vi "明场校正.vi"() -> ()   [LabVIEW 2018]
uses:
  <vilib>/vision/Process.llb/Surface Fit Options.ctl
  <vilib>/vision/Process.llb/Background Estimation Options.ctl
  <vilib>/vision/NI_Vision_Development_Module.lvlib
panel:
  in  "停止":bool
  out "error out":errorcluster
  out "Image":T1(plugin-control)
  in  "枚举":enum16{"估算", "采集"}(ring)
  in  "Background Estimation Options":T2={"Estimate Background?"=FALSE, "Method"=0, "Polynomial Degree"=2, "Window Size (32x32)"={"SizeX"=32, "SizeY"=32}, "Niblack Deviation Factor (0.2)"=0.2} {"Niblack Deviation Factor (0.2)" min=0.0 max=1.0 format="%.2f"; "Window Size (32x32)"."SizeY" min=3 step=1; "Window Size (32x32)"."SizeX" min=3 step=1; "Method" items=["Polynomial", "Background Correction", "NiBlack"]}
  in  "Surface Fit Options":T3={"Model"=0, "Sampling Grid Size"={"SizeX"=100, "SizeY"=100}, "Polynomial Degree"=2} {"Sampling Grid Size"."SizeY" min=3 step=1; "Sampling Grid Size"."SizeX" min=3 step=1; "Model" items=["Polynomial"]}
  in  "路径":path
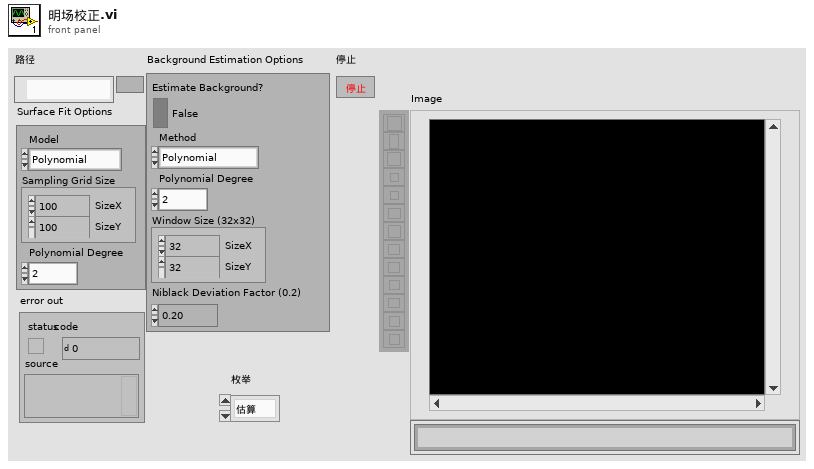
[diagram p1: front panel]
types:
  T1 = typedef "IMAQ Image.ctl" = refnum<image>
  T2 = typedef "Background Estimation Options.ctl" = cluster{"Estimate Background?":bool, "Method":i32, "Polynomial Degree":i32, "Window Size (32x32)":cluster{"SizeX":i32, "SizeY":i32}, "Niblack Deviation Factor (0.2)":dbl}
  T3 = typedef "Surface Fit Options.ctl" = cluster{"Model":i32, "Sampling Grid Size":cluster{"SizeX":i32, "SizeY":i32}, "Polynomial Degree":i32}
  T4 = cluster{"Surface Fit Options":T3, "Background Estimation Options":T2, "枚举":enum16{"估算", "采集"}}
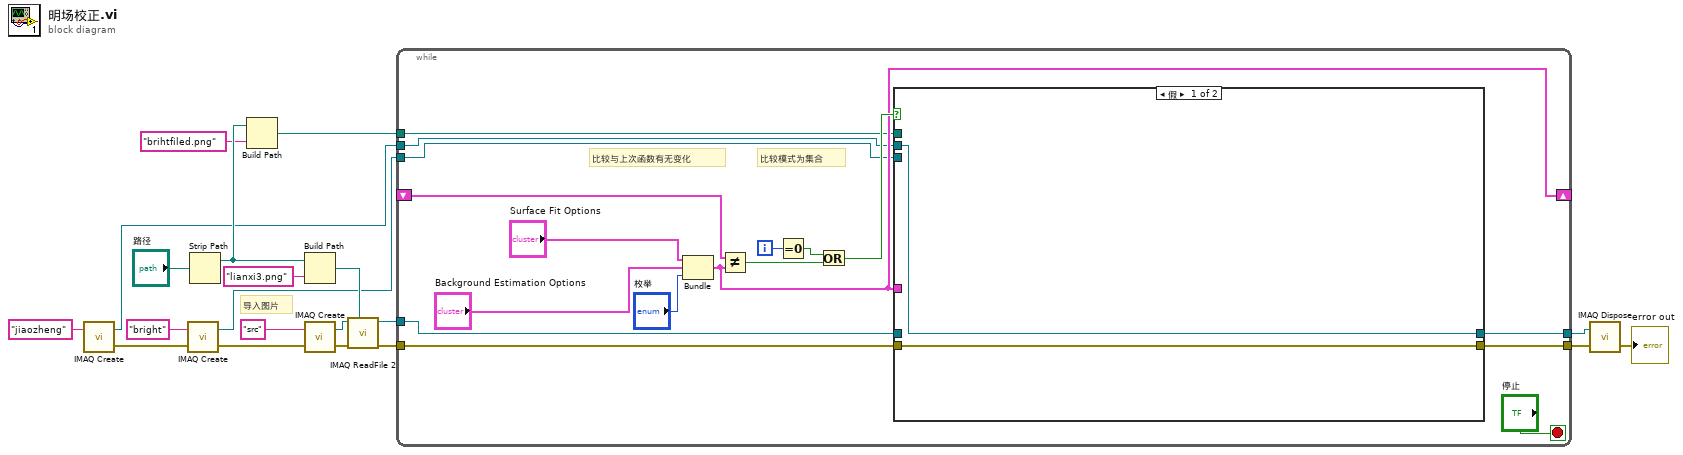
[diagram p0: block diagram]
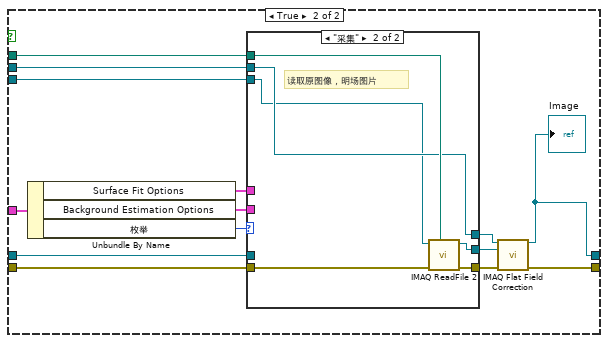
[diagram p2: hidden frame]
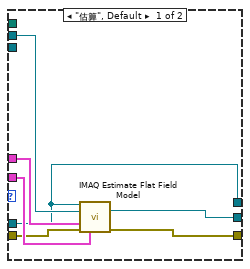
[diagram p3: hidden frame]
diagram:
  # "导入图片"
  n1 = call "IMAQ Create"("Image Name"="jiaozheng") -> ("New Image"=w11:T1, "error out"=w2:errorcluster)  [unwired: 4 in]
  n2 = call "IMAQ Create"("Image Name"="bright", "error in (no error)"=w2) -> ("New Image"=w4:T1, "error out"=w3:errorcluster)  [unwired: 3 in]
  n3 = Strip Path(path="路径") -> (stripped path=w19:path)  [unwired: 1 out]
  n4 = Build Path(base path=w19, name or relative path="brihtfiled.png" ("名称或相对路径")) -> (appended path=w6:path)
  n5 = Build Path(base path=w19, name or relative path="lianxi3.png" ("名称或相对路径")) -> (appended path=w15:path)
  n6 = call "IMAQ Create"("Image Name"="src", "error in (no error)"=w3) -> ("New Image"=w14:T1, "error out"=w13:errorcluster)  [unwired: 3 in]
  n7 = call "IMAQ ReadFile 2"("File Path"=w15, "error in (no error)"=w13, "Image"=w14) -> ("error out"=w10:errorcluster, "Image Out"=w12:T1)  [unwired: 4 in, 3 out]
  n8 = while {
    shift-right: [w29] -> _
    shift-left: _ -> [w34]
    tunnel: w12 -> [w28]
    tunnel: w11 -> [w27]
    tunnel: w10 -> [w26]
    tunnel: [w25] -> w9
    tunnel: [w24] -> w8
    tunnel: w6 -> [w23]
    tunnel: w4 -> [w22]
    i -> [w33]
    stop <- "停止" stop-if-true
    # "比较模式为集合"
    # "比较与上次函数有无变化"
    n9 = Bundle("Surface Fit Options"="Surface Fit Options", "Background Estimation Options"="Background Estimation Options", "枚举"="枚举") -> (w29:T4)  [unwired: 1 in]
    n10 = Not Equal?(x=w34, y=w29) -> (x != y?=w31:bool)
    n11 = Equal To 0?(x=w33) -> (x = 0?=w32:bool)
    n12 = Or(x=w32, y=w31) -> (x .or. y?=w30:bool)
    n13 = case shown="假" w30 {
      tunnel: w29 -> [_ w53]
      tunnel: w28 -> [_ w51]
      tunnel: w27 -> [w38 w48]
      tunnel: w26 -> [w39 w47]
      tunnel: [w38 w43] -> w25
      tunnel: [w39 w42] -> w24
      tunnel: w23 -> [_ w41]
      tunnel: w22 -> [_ w40]
      frame False {
      }
      frame True {
        n14 = Unbundle By Name(w53) -> ("Surface Fit Options"=w50:T3, "Background Estimation Options"=w49:T2, "枚举"=w52:enum16{"估算", "采集"})
        n15 = case shown="\"采集\"" w52 {
          tunnel: w51 -> [w56 _]
          tunnel: w50 -> [w60 _]
          tunnel: w49 -> [w59 _]
          tunnel: w48 -> [w58 w63]
          tunnel: w47 -> [w57 w61]
          tunnel: [w56 w63] -> w46
          tunnel: [w55 w64] -> w45
          tunnel: [w54 w65] -> w44
          tunnel: w41 -> [_ w66]
          tunnel: w40 -> [_ w62]
          frame "估算", Default {
            n16 = call "IMAQ Estimate Flat Field Model"("Image Src"=w56, "Image Dst"=w58, "Surface Fit Options"=w60, "error in (no error)"=w57, "Background Estimation Options"=w59) -> ("Flat Field Image Out"=w55:T1, "error out"=w54:errorcluster)  [unwired: 9 in]
          }
          frame "采集" {
            # "读取原图像，明场图片"
            n17 = call "IMAQ ReadFile 2"("File Path"=w66, "error in (no error)"=w61, "Image"=w62) -> ("error out"=w65:errorcluster, "Image Out"=w64:T1)  [unwired: 4 in, 3 out]
          }
        }
        n18 = call "IMAQ Flat Field Correction"("Image Src"=w46, "Image Dst"=w45, "error in (no error)"=w44) -> ("Corrected Image"=w43:T1, "error out"=w42:errorcluster)  [unwired: 10 in, 1 out]
        "Image" <- w43
      }
    }
  }
  n19 = call "IMAQ Dispose"("Image"=w9, "error in (no error)"=w8) -> ("error out"=→"error out":errorcluster)  [unwired: 4 in]
